vi "Modbus Config File Path.vi"(11 "appended path in":path) -> (3 "appended path out":path)   [LabVIEW 2021]
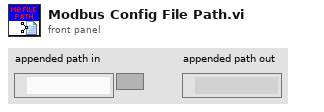
[diagram p1: front panel]
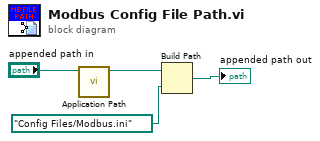
[diagram p0: block diagram]
diagram:
  n1 = call "Application Path.vi"("name or relative path"="appended path in") -> ("appended path"=w4:path)  [unwired: 10 in]
  n2 = Build Path(base path=w4, name or relative path=path "Config Files/Modbus.ini") -> (appended path=→"appended path out":path)
